vi "Threshold_Mass_Flow_Rate.vi"(6 "higher threshold":dbl, 9 "Primary Flow\n\n\nFM-40 [kg/s]":sgl, 10 "lower threshold":dbl, 11 "Digital in":refnum<vi>) -> ()   [LabVIEW 2017]
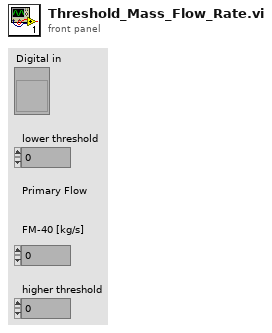
[diagram p1: front panel]
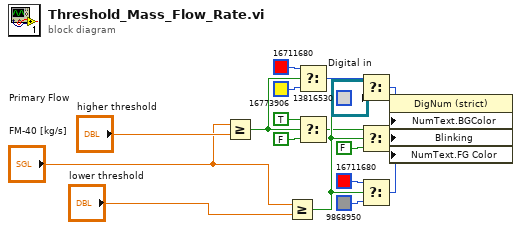
[diagram p0: block diagram]
diagram:
  n1 = Greater Or Equal?(x="Primary Flow\n\n\nFM-40 [kg/s]", y="higher threshold") -> (x >= y?=w18:bool)
  n2 = Greater Or Equal?(x="Primary Flow\n\n\nFM-40 [kg/s]", y="lower threshold") -> (x >= y?=w19:bool)
  n3 = Select(t=u32 16711680, s=w18, f=u32 16773906) -> (s? t:f=w4:u32)
  n4 = Select(t=TRUE ("Blinking"), s=w18, f=FALSE ("Blinking")) -> (s? t:f=w13:bool)
  n5 = Select(t=w4, s=w19, f=u32 13816530) -> (s? t:f=w9:u32)
  n6 = Select(t=w13, s=w19, f=FALSE ("Blinking")) -> (s? t:f=w14:bool)
  n7 = Select(t=u32 16711680, s=w19, f=u32 9868950) -> (s? t:f=w17:u32)
  n8 = property on="Property Node" class="DigNum (strict)"(reference="Digital in", "NumText.BGColor"=w9, "Blinking"=w14, "NumText.FG Color"=w17) -> ()  [unwired: 1 in, 2 out]
